vi "Path manager.vi"(3 "error in":errorcluster, 4 "File Type":string=".bat", 5 "File Path":path=path "E:/Mechmet Engineers/Test run results") -> (0 "error out":errorcluster, 2 "refnum out":refnum<file>)   [LabVIEW 2024]
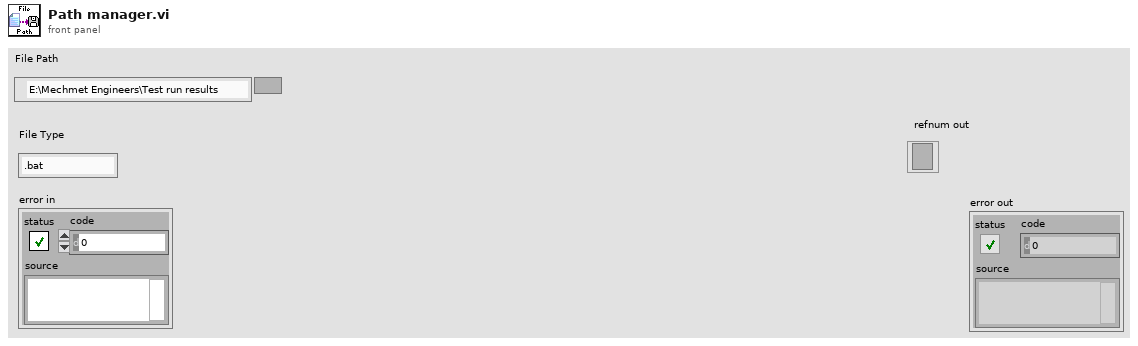
[diagram p1: front panel]
types:
  T1 = enum16{"open", "replace", "create", "open or create", "replace or create", "replace or create with confirmation"}
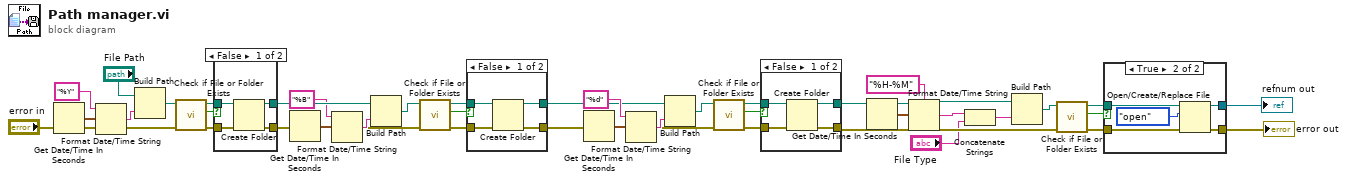
[diagram p0: block diagram]
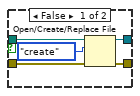
[diagram p3: hidden frame]
diagram:
  n1 = Get Date/Time In Seconds() -> (seconds since 1Jan1904=w20:timestamp)
  n2 = Format Date/Time String(time format string (%c)="%Y", seconds (now)=w20) -> (date/time string=w22:string)  [unwired: 1 in]
  n3 = Build Path(base path="File Path", name or relative path=w22) -> (appended path=w21:path)
  n4 = call <vilib>:"Check if File or Folder Exists.vi"("error in (no error)"="error in", "path"=w21) -> ("error out"=w26:errorcluster, "file or folder exists?"=w24:bool, "dup path"=w25:path)  [unwired: 7 in]
  n5 = case shown="False" w24 {
    tunnel: w25 -> [w41 w46]
    tunnel: [w43 w46] -> w30
    tunnel: [w42 w45] -> w28
    tunnel: w26 -> [w44 w45]
    frame False {
      n6 = Create Folder(path (use dialog)=w41, error in=w44) -> (created path=w43:path, error out=w42:errorcluster)  [unwired: 1 in, 1 out]
    }
    frame True {
    }
  }
  n7 = Get Date/Time In Seconds() -> (seconds since 1Jan1904=w29:timestamp)
  n8 = Format Date/Time String(time format string (%c)="%B", seconds (now)=w29) -> (date/time string=w31:string)  [unwired: 1 in]
  n9 = Build Path(base path=w30, name or relative path=w31) -> (appended path=w32:path)
  n10 = call <vilib>:"Check if File or Folder Exists.vi"("error in (no error)"=w28, "path"=w32) -> ("error out"=w34:errorcluster, "file or folder exists?"=w18:bool, "dup path"=w33:path)  [unwired: 7 in]
  n11 = case shown="False" w18 {
    tunnel: w33 -> [w47 w52]
    tunnel: [w49 w52] -> w2
    tunnel: [w48 w51] -> w3
    tunnel: w34 -> [w50 w51]
    frame False {
      n12 = Create Folder(path (use dialog)=w47, error in=w50) -> (created path=w49:path, error out=w48:errorcluster)  [unwired: 1 in, 1 out]
    }
    frame True {
    }
  }
  n13 = Get Date/Time In Seconds() -> (seconds since 1Jan1904=w8:timestamp)
  n14 = Format Date/Time String(time format string (%c)="%d", seconds (now)=w8) -> (date/time string=w7:string)  [unwired: 1 in]
  n15 = Build Path(base path=w2, name or relative path=w7) -> (appended path=w6:path)
  n16 = call <vilib>:"Check if File or Folder Exists.vi"("error in (no error)"=w3, "path"=w6) -> ("error out"=w4:errorcluster, "file or folder exists?"=w9:bool, "dup path"=w5:path)  [unwired: 7 in]
  n17 = case shown="False" w9 {
    tunnel: w5 -> [w53 w58]
    tunnel: [w55 w58] -> w1
    tunnel: [w54 w57] -> w40
    tunnel: w4 -> [w56 w57]
    frame False {
      n18 = Create Folder(path (use dialog)=w53, error in=w56) -> (created path=w55:path, error out=w54:errorcluster)  [unwired: 1 in, 1 out]
    }
    frame True {
    }
  }
  n19 = Get Date/Time In Seconds() -> (seconds since 1Jan1904=w35:timestamp)
  n20 = Format Date/Time String(time format string (%c)="%H-%M", seconds (now)=w35) -> (date/time string=w12:string)  [unwired: 1 in]
  n21 = Concatenate Strings(w12, "File Type") -> (w13:string)
  n22 = Build Path(base path=w1, name or relative path=w13) -> (appended path=w36:path)
  n23 = call <vilib>:"Check if File or Folder Exists.vi"("error in (no error)"=w40, "path"=w36) -> ("error out"=w38:errorcluster, "file or folder exists?"=w39:bool, "dup path"=w37:path)  [unwired: 7 in]
  n24 = case shown="True" w39 {
    tunnel: w37 -> [w59 w64]
    tunnel: [w62 w67] -> w16
    tunnel: [w61 w66] -> w17
    tunnel: w38 -> [w63 w68]
    frame False {
      n25 = Open/Create/Replace File(file path (use dialog)=w59, error in=w63, operation (0:open)=T1."create") -> (refnum out=w62:refnum<file>, error out=w61:errorcluster)  [unwired: 3 in, 1 out]
    }
    frame True {
      n26 = Open/Create/Replace File(file path (use dialog)=w64, error in=w68, operation (0:open)=T1."open") -> (refnum out=w67:refnum<file>, error out=w66:errorcluster)  [unwired: 3 in, 1 out]
    }
  }
  "error out" <- w17
  "refnum out" <- w16
